vi "ParseArgumentsCore.vi"(8 "error in (no error)":errorcluster, 10 "Inputs":string[](array[string]), 11 "RunUnitTests in":refnum<class "RunUnitTests.lvclass">) -> (0 "error out":errorcluster, 3 "RunUnitTests out":refnum<class "RunUnitTests.lvclass">)   [LabVIEW 2014, in "RunUnitTests.lvclass"]
uses:
  RunUnitTests.lvclass
  RunUnitTests.lvclass/RunUnitTests.ctl
  Utilities/OperationErrorType.ctl
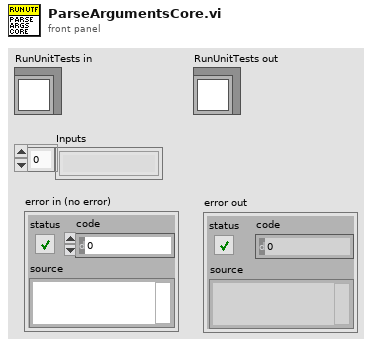
[diagram p1: front panel]
types:
  T1 = typedef "OperationErrorType.ctl" = enum16{"RequiredArgumentMissing", "UnknownArguments", "LoggerSetMultipleTimes", "OperationBrokenError"}
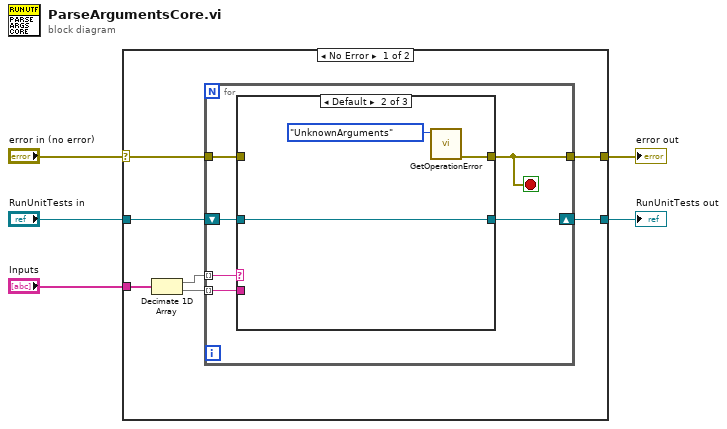
[diagram p0: block diagram]
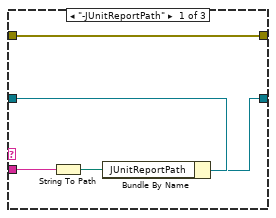
[diagram p2: hidden frame]
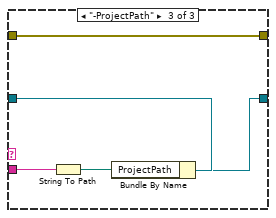
[diagram p3: hidden frame]
diagram:
  n1 = case shown="No Error" "error in (no error)" {
    selector: "error in (no error)" -> [w6 w33]
    tunnel: [w12 w32] -> w5
    tunnel: "RunUnitTests in" -> [w11 w32]
    tunnel: "Inputs" -> [w8 _]
    tunnel: [w7 w33] -> w1
    frame No Error {
      n2 = Decimate 1D Array(w8) -> (w9:string[], w10:string[])
      n3 = for {
        tunnel: w9 -> [w18] mode=indexing
        tunnel: w10 -> [w15] mode=indexing
        shift-right: [w16] -> w12
        shift-left: w11 -> [w17]
        tunnel: [w13] -> w7
        tunnel: w6 -> [w14]
        stop <- w13 stop-if-true
        n4 = case shown="Default" w18 {
          tunnel: w17 -> [w23 w26 w31]
          tunnel: [w22 w26 w30] -> w16
          tunnel: w15 -> [w20 _ w28]
          tunnel: [w19 w25 w27] -> w13
          tunnel: w14 -> [w19 _ w27]
          frame "-JUnitReportPath" {
            n5 = String To Path(string=w20) -> (path=w21:path)
            n6 = Bundle By Name(cluster=w23, "JUnitReportPath"=w21) -> (w22:refnum<class "RunUnitTests.lvclass">)
          }
          frame Default {
            n7 = call "GetOperationError.vi"("Operation Error Type"=OperationErrorType."UnknownArguments") -> ("error out"=w25:errorcluster)  [unwired: 10 in]
          }
          frame "-ProjectPath" {
            n8 = String To Path(string=w28) -> (path=w29:path)
            n9 = Bundle By Name(cluster=w31, "ProjectPath"=w29) -> (w30:refnum<class "RunUnitTests.lvclass">)
          }
        }
      }
    }
    frame Error {
    }
  }
  "RunUnitTests out" <- w5
  "error out" <- w1
